vi "ParseNumeric.vi"(11 "String In":string) -> (3 "Numeric":u32)   [LabVIEW 2019, in "A2L Utility.lvlib"]
uses:
  A2L Utility.lvlib
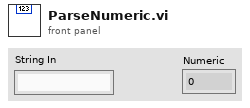
[diagram p1: front panel]
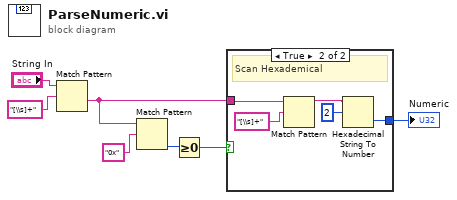
[diagram p0: block diagram]
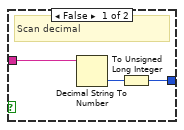
[diagram p2: hidden frame]
diagram:
  n1 = Match Pattern(string="String In", regular expression="[\\s]+") -> (after substring=w2:string)  [unwired: 1 in, 3 out]
  n2 = Match Pattern(string=w2, regular expression="0x") -> (offset past match=w5:i32)  [unwired: 1 in, 3 out]
  n3 = Greater Or Equal To 0?(x=w5) -> (x >= 0?=w4:bool)
  n4 = case shown="True" w4 {
    tunnel: w2 -> [w10 w15]
    tunnel: [w8 w12] -> w7
    frame False {
      # "Scan decimal"
      n5 = Decimal String To Number(string=w10) -> (number=w9:i32)  [unwired: 2 in, 1 out]
      n6 = To Unsigned Long Integer(number=w9) -> (unsigned 32bit integer=w8:u32)
    }
    frame True {
      # "Scan Hexademical"
      n7 = Match Pattern(string=w15, regular expression="[\\s]+") -> (before substring=w14:string)  [unwired: 1 in, 3 out]
      n8 = Hexadecimal String To Number(string=w14, offset=2) -> (number=w12:u32)  [unwired: 1 in, 1 out]
    }
  }
  "Numeric" <- w7
